vi "SDI Test Suite - MAIN.vi"() -> ()   [LabVIEW 2014]
uses:
  Controls/States.ctl
  <vilib>/Motion/Express/_s/nimc.ex.straightLineMove.startStraightLineMove.axis.modeRelative.0.vi
  <vilib>/Motion/plugins/PluginFramework/nismPluginAxisBase/nismPluginAxisBaseClass.lvclass
  <vilib>/Motion/BlockNode/FB.NIMotion.xnode
  C:/Users/mpool/Documents/LabVIEW Data/Untitled Project 3/Template SoftMotion Drive Interface Plug-in Class.lvclass
  <resource>/objmgr/nimcca.rc
panel:
  out "Straight Line Result":T1
  in  "Path to Open.vi not listed (Optional)":path
  in  "Axis":refnum<k21>
  in  "Boolean":bool
  in  "Listbox":i32(listbox)
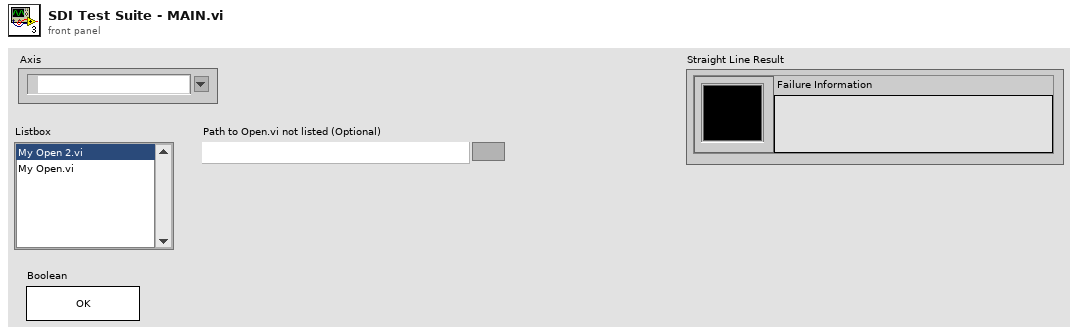
[diagram p1: front panel]
types:
  T1 = cluster{"Straight Line Result":u32, "Failure Information":string}
  T2 = typedef "States.ctl" = enum16{"Initialize", "Insert Open VI", "Run Open VI", "Straight Line", "Home", "Limit", "Generate Report", "Finalize", "Terminate"}
  T3 = enum8{"Enabled", "Disabled", "Disabled and Grayed Out"}
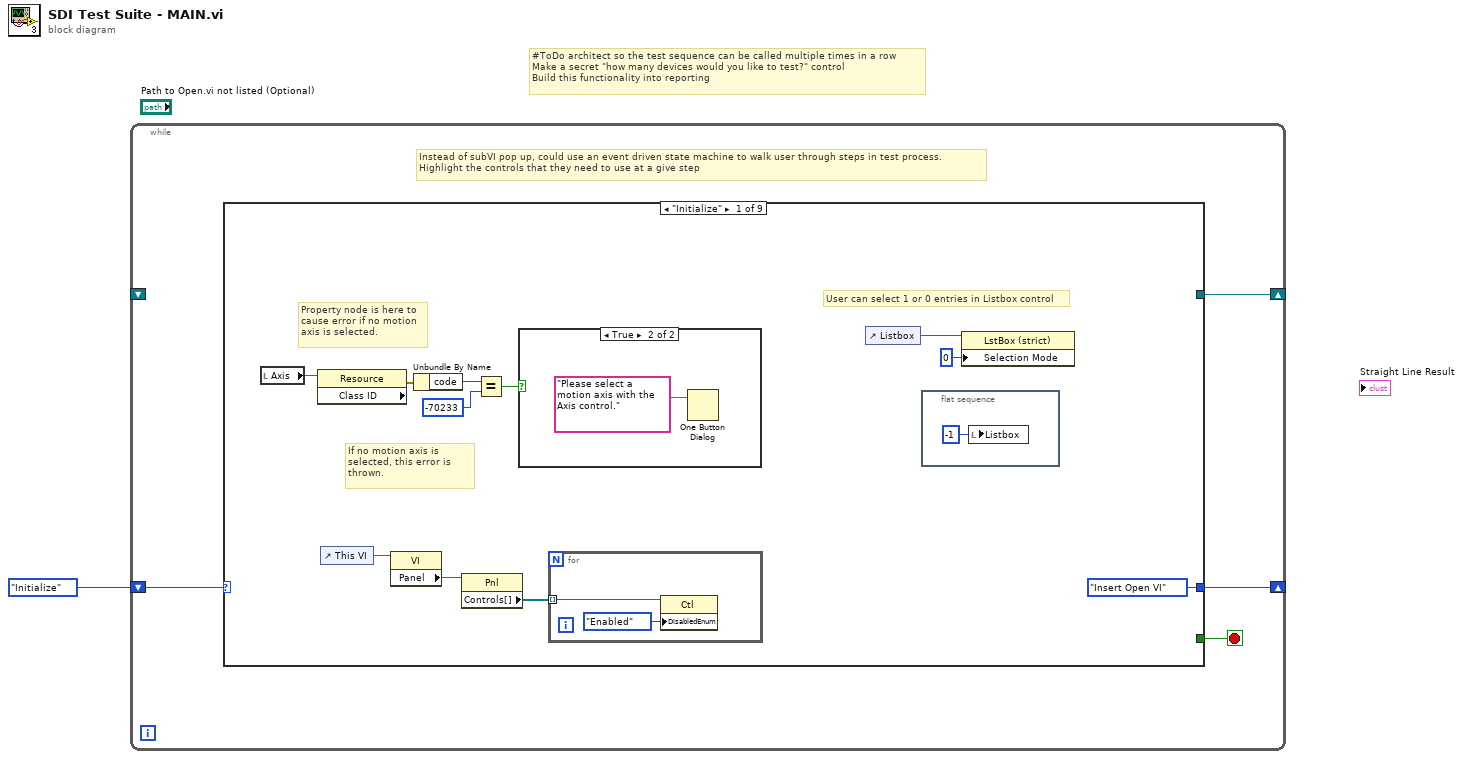
[diagram p0: block diagram]
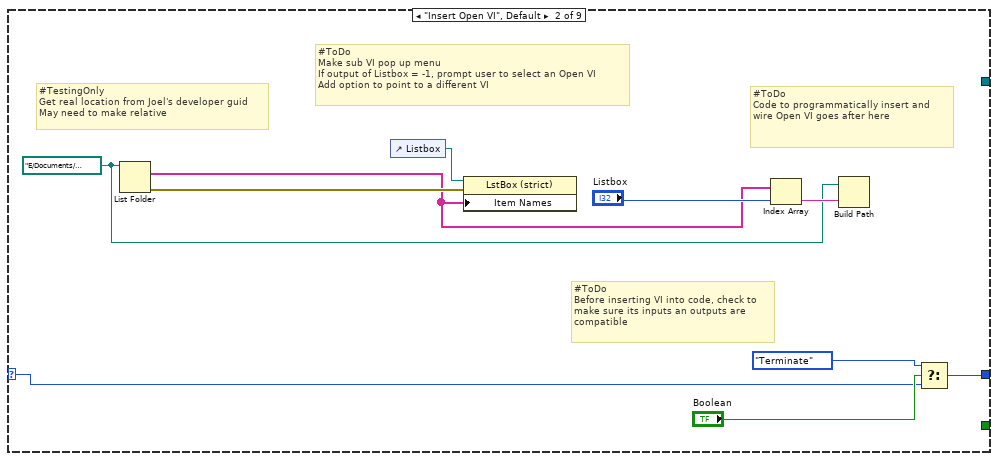
[diagram p3: hidden frame]
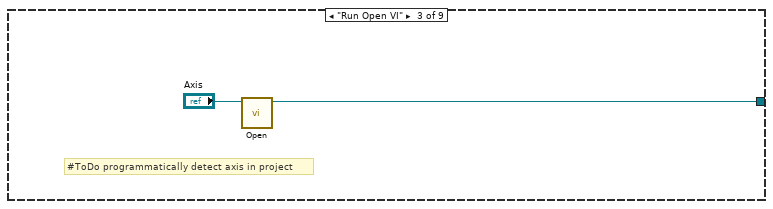
[diagram p4: hidden frame]
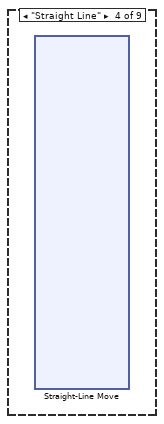
[diagram p5: hidden frame]
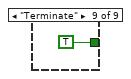
[diagram p10: hidden frame]
diagram:
  # "#ToDo architect so the test sequence can be called multiple times in a row\nMake a secret \"how many devices would you like to test?\" control\nBuild this functionality into reporting"
  n1 = while {
    shift-right: [w3] -> _
    shift-left: States."Initialize" -> [w5]
    shift-right: [w2] -> _
    shift-left: _ -> [_]
    stop <- w4 stop-if-true
    # "Instead of subVI pop up, could use an event driven state machine to walk user through steps in test process.\nHighlight the controls that they need to use at a give step"
    n2 = case shown="\"Initialize\"" w5 {
      selector: w5 -> [_ w26 _ _ _ _ _ _ _]
      tunnel: [_ _ _ _ _ _ _ _ TRUE] -> w4
      tunnel: [States."Insert Open VI" w30 _ _ _ _ _ _ _] -> w3
      tunnel: [_ _ w31 _ _ _ _ _ _] -> w2
      frame "Initialize" {
        # "If no motion axis is selected, this error is thrown."
        # "User can select 1 or 0 entries in Listbox control"
        # "Property node is here to cause error if no motion axis is selected."
        n3 = local read "Axis"() -> (w13:refnum<k21>)
        n4 = property class="Resource" props=["Class ID"](reference=w13) -> (error out=w12:errorcluster)  [unwired: 1 in, 2 out]
        n5 = control-ref of="This VI"() -> (w8:refnum<vi>)
        n6 = property class="VI"(reference=w8) -> ("Panel"=w7:refnum<vi>)  [unwired: 1 in, 2 out]
        n7 = Unbundle By Name(w12) -> ("code"=w11:i32)
        n8 = property class="Pnl"(reference=w7) -> ("Controls[]"=w6:refnum<vi>[])  [unwired: 1 in, 2 out]
        n9 = Equal?(x=w11, y=-70233) -> (x = y?=w9:bool)
        n10 = case shown="True" w9 {
          frame False {
          }
          frame True {
            n11 = One Button Dialog(message="Please select a motion axis with the Axis control.") -> ()  [unwired: 1 in, 1 out]
          }
        }
        n12 = for {
          tunnel: w6 -> [w17] mode=indexing
          n13 = property class="Ctl"(reference=w17, "DisabledEnum"=T3."Enabled" ("Disabled")) -> ()  [unwired: 1 in, 2 out]
        }
        n14 = control-ref of="Listbox"() -> (w15:refnum<vi>)
        n15 = flat-sequence {
          frame #0 {
            n16 = local write "Listbox"(-1 ("Listbox")) -> ()
          }
        }
        n17 = property class="LstBox (strict)"(reference=w15, "Selection Mode"=0) -> ()  [unwired: 1 in, 2 out]
      }
      frame "Insert Open VI", Default {
        w22 = path "E:/Documents/Projects/Projects on GitHub/SDI Test Suite/Test" ("path")
        # "#ToDo\nBefore inserting VI into code, check to make sure its inputs an outputs are compatible"
        # "#ToDo\nCode to programmatically insert and wire Open VI goes after here"
        # "#ToDo\nMake sub VI pop up menu\nIf output of Listbox = -1, prompt user to select an Open VI\nAdd option to point to a different VI"
        # "#TestingOnly\nGet real location from Joel's developer guid\nMay need to make relative"
        n18 = List Folder(path=w22) -> (filenames=w21:string[], error out=w25:errorcluster)  [unwired: 3 in, 2 out]
        n19 = control-ref of="Listbox"() -> (w29:refnum<vi>)
        n20 = property class="LstBox (strict)"(reference=w29, error in=w25, "Item Names"=w21) -> ()  [unwired: 2 out]
        n21 = Index Array(array=w21, index="Listbox") -> (element=w23:string)
        n22 = Build Path(base path=w22, name or relative path=w23) -> ()  [unwired: 1 out]
        n23 = Select(t=States."Terminate" ("f"), s="Boolean", f=w26) -> (s? t:f=w30:T2)
      }
      frame "Run Open VI" {
        # "#ToDo programmatically detect axis in project"
        n24 = call "Open.vi"("Axis"="Axis") -> ("Base Axis Out"=w31:refnum<class "nismPluginAxisBaseClass.lvclass">)  [unwired: 9 in, 1 out]
      }
      frame "Straight Line" {
        n25 = xnode ("Straight-Line Move")() -> ()  [unwired: 10 in, 3 out]
      }
      frame "Home" {
      }
      frame "Limit" {
      }
      frame "Generate Report" {
      }
      frame "Finalize" {
      }
      frame "Terminate" {
      }
    }
  }
